vi "ScanWrapper.vi"(7 "format string":string="%f", 8 "error in (no error)":errorcluster, 9 "default value 1":dbl=nan, 10 "initial scan location":u32, 11 "input string":string) -> (0 "error out":errorcluster, 1 "output 1":dbl, 2 "offset past scan":u32, 3 "remaining string":string, 4 "No number found":bool)   [LabVIEW 2018]
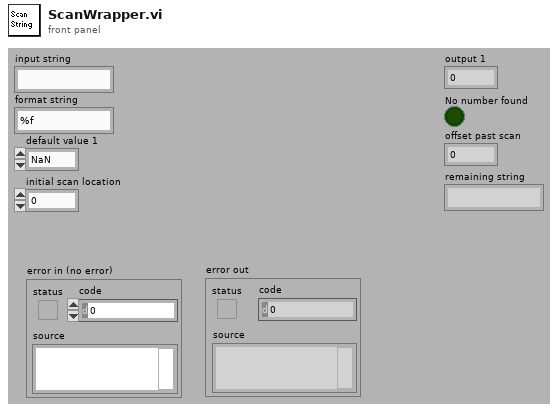
[diagram p1: front panel]
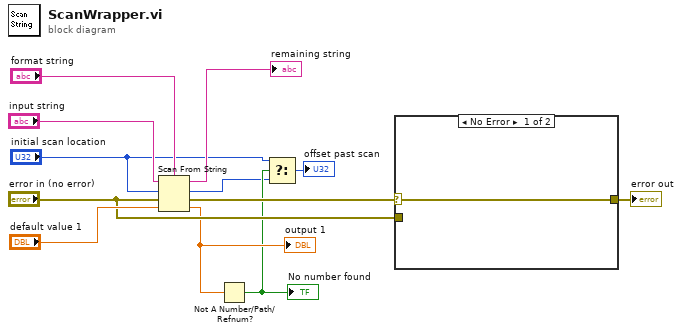
[diagram p0: block diagram]
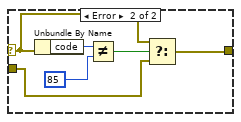
[diagram p2: hidden frame]
diagram:
  n1 = Scan From String(format string="format string", input string="input string", initial scan location="initial scan location", error in="error in (no error)", default 1="default value 1") -> (remaining string=→"remaining string":string, offset past scan=w3:u32, error out=w8:errorcluster, output 1=w5:dbl)
  "output 1" <- w5
  n2 = Not A Number/Path/Refnum?(number/path/refnum=w5) -> (NaN/Path/Refnum?=w4:bool)
  "No number found" <- w4
  n3 = Select(t="initial scan location", s=w4, f=w3) -> (s? t:f=→"offset past scan":u32)
  n4 = case shown="No Error" w8 {
    selector: w8 -> [w13 w15]
    tunnel: "error in (no error)" -> [_ w16]
    tunnel: [w13 w14] -> w6
    frame No Error {
    }
    frame Error {
      n5 = Unbundle By Name(w15) -> ("code"=w19:i32)
      n6 = Not Equal?(x=w19, y=85 ("code")) -> (x != y?=w17:bool)
      n7 = Select(t=w15, s=w17, f=w16) -> (s? t:f=w14:errorcluster)
    }
  }
  "error out" <- w6
